vi "BASECMD.vi"(8 "PARÁMETRO 2":string, 9 "PARÁMETRO 1":string, 10 "COMANDOS":T1, 11 "MICROS":T2) -> (3 "COMANDO":string)   [LabVIEW 2019, in "SERIAL DEVICE.lvclass"]
uses:
  SERIAL DEVICE.lvclass
  MICROS.ctl
  COMANDOS.ctl
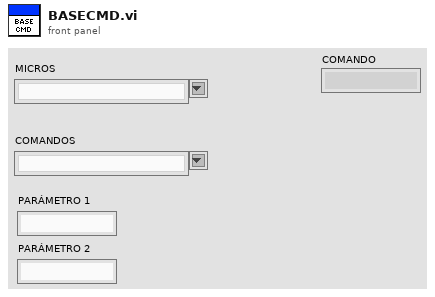
[diagram p1: front panel]
types:
  T1 = typedef "COMANDOS.ctl" = string
  T2 = typedef "MICROS.ctl" = string
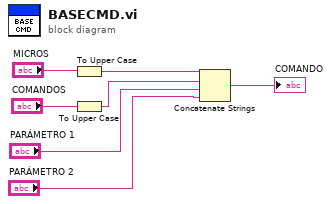
[diagram p0: block diagram]
diagram:
  n1 = To Upper Case(1:"MICROS") -> (0:w6:T2)
  n2 = To Upper Case(1:"COMANDOS") -> (0:w4:T1)
  n3 = Concatenate Strings(w6, w4, "PARÁMETRO 1", "PARÁMETRO 2") -> (→"COMANDO":string)
